vi "Range to OHM Span.vi"(5 "Range And Span":T1={"OHM Range (0 : 20ohm)"=0, "Enable Span (False)"=FALSE, "Lower Span (0.000ohm)"=0.0, "Upper Span (20.000ohm)"=20.0, "Bias (0)"=0.0} {"Upper Span (20.000ohm)" min=-99999.0 max=99999.0 step=1.0 format="%_5g"; "Lower Span (0.000ohm)" min=-99999.0 max=99999.0 step=1.0 format="%_5g"; "OHM Range (0 : 20ohm)" items=["20ohm", "200ohm", "2000ohm"]}, 7 "Scaling? (False)":bool, 9 "Floating Point Position (2)":i32=2) -> (6 "Lower Span":i32 min=-99999 max=99999 step=1, 8 "Upper Span":i32=20 min=-99999 max=99999 step=1, 10 "Bias":i32)   [LabVIEW 2020, in "Yokogawa GX Series.lvlib"]
doc: "This VI gets the OHM span value from the range."
uses:
  <instrlib>/Yokogawa GX Series/Yokogawa GX Series.lvlib
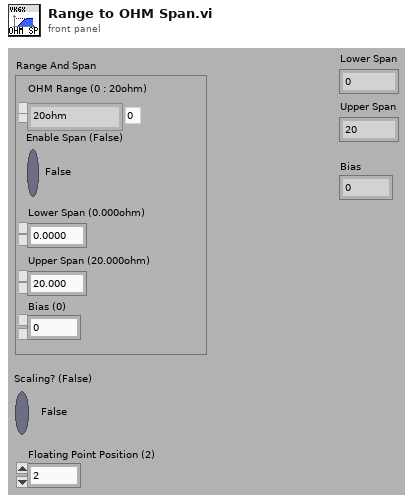
[diagram p1: front panel]
types:
  T1 = cluster{"OHM Range (0 : 20ohm)":i32, "Enable Span (False)":bool, "Lower Span (0.000ohm)":dbl, "Upper Span (20.000ohm)":dbl, "Bias (0)":dbl}
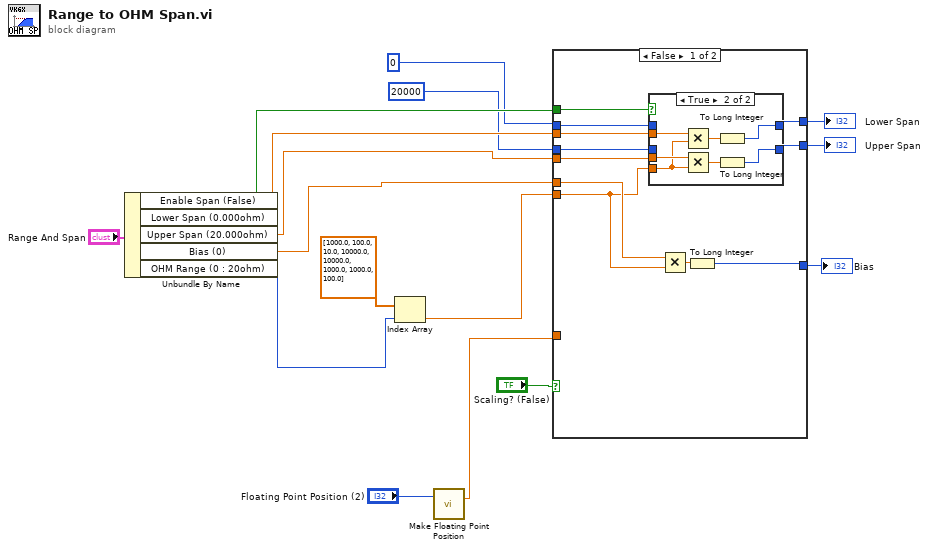
[diagram p0: block diagram]
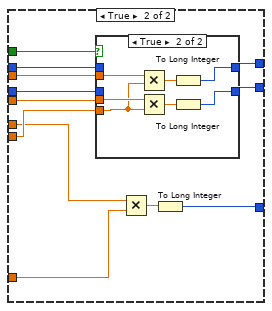
[diagram p3: hidden frame]
diagram:
  n1 = Unbundle By Name("Range And Span") -> ("Enable Span (False)"=w7:bool, "Lower Span (0.000ohm)"=w8:dbl, "Upper Span (20.000ohm)"=w9:dbl, "Bias (0)"=w10:dbl, "OHM Range (0 : 20ohm)"=w11:i32)
  n2 = Index Array(array=dbl[] [1000.0, 100.0, 10.0, 10000.0, 10000.0, 1000.0, 1000.0, 100.0], index=w11) -> (element=w16:dbl)
  n3 = call <instrlib>:"Make Floating Point Position.vi"("Floating Point Position (2)"="Floating Point Position (2)") -> ("Times"=w3:dbl)  [unwired: 14 in]
  n4 = case shown="False" "Scaling? (False)" {
    tunnel: w16 -> [w17 w41]
    tunnel: 0 -> [w27 w48]
    tunnel: 20000 -> [w26 w47]
    tunnel: [w25 w46] -> w15
    tunnel: [w24 w45] -> w14
    tunnel: [w19 w37] -> w12
    tunnel: w10 -> [w18 w38]
    tunnel: w9 -> [w23 w44]
    tunnel: w8 -> [w22 w43]
    tunnel: w7 -> [w21 w42]
    tunnel: w3 -> [_ w39]
    frame False {
      n5 = case shown="True" w21 {
        tunnel: w22 -> [_ w35]
        tunnel: w23 -> [_ w34]
        tunnel: [w29 w32] -> w25
        tunnel: [w28 w31] -> w24
        tunnel: w27 -> [w29 _]
        tunnel: w26 -> [w28 _]
        tunnel: w17 -> [_ w30]
        frame False {
        }
        frame True {
          n6 = Multiply(x=w35, y=w30) -> (x*y=w36:dbl)
          n7 = Multiply(x=w34, y=w30) -> (x*y=w33:dbl)
          n8 = To Long Integer(number=w36) -> (32bit integer=w32:i32)
          n9 = To Long Integer(number=w33) -> (32bit integer=w31:i32)
        }
      }
      n10 = Multiply(x=w18, y=w17) -> (x*y=w20:dbl)
      n11 = To Long Integer(number=w20) -> (32bit integer=w19:i32)
    }
    frame True {
      n12 = case shown="True" w42 {
        tunnel: w43 -> [_ w56]
        tunnel: w44 -> [_ w55]
        tunnel: [w50 w53] -> w46
        tunnel: [w49 w52] -> w45
        tunnel: w48 -> [w50 _]
        tunnel: w47 -> [w49 _]
        tunnel: w41 -> [_ w51]
        frame False {
        }
        frame True {
          n13 = Multiply(x=w56, y=w51) -> (x*y=w57:dbl)
          n14 = Multiply(x=w55, y=w51) -> (x*y=w54:dbl)
          n15 = To Long Integer(number=w57) -> (32bit integer=w53:i32)
          n16 = To Long Integer(number=w54) -> (32bit integer=w52:i32)
        }
      }
      n17 = Multiply(x=w38, y=w39) -> (x*y=w40:dbl)
      n18 = To Long Integer(number=w40) -> (32bit integer=w37:i32)
    }
  }
  "Lower Span" <- w15
  "Upper Span" <- w14
  "Bias" <- w12
